vi "live open.vi"(8 "error in (no error)":errorcluster, 11 "DAQCascade512II":refnum<class "DAQCascade512II.lvclass">) -> (0 "error out":errorcluster, 3 "DAQCascade512II out":refnum<class "DAQCascade512II.lvclass">)   [LabVIEW 2012, in "DAQCascade512II.lvclass"]
uses:
  DAQCascade512II.lvclass
  DAQCascade512II.lvclass/DAQCascade512II.ctl
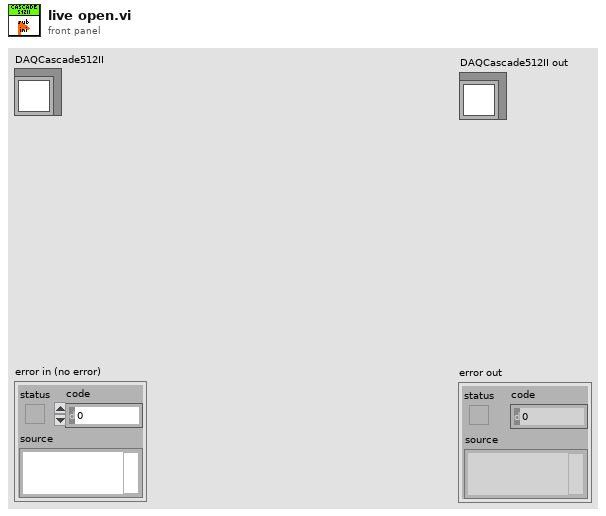
[diagram p1: front panel]
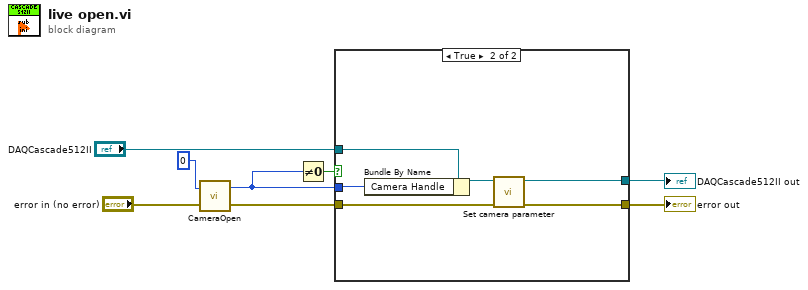
[diagram p0: block diagram]
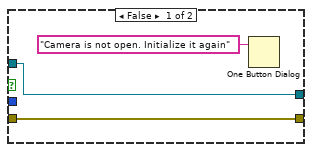
[diagram p2: hidden frame]
diagram:
  n1 = call <userlib>:"CameraOpen.vi"("error in"="error in (no error)", "Camera Device ID"=u32 0) -> ("error out"=w3:errorcluster, "Camera Handle"=w1:u32)
  n2 = Not Equal To 0?(x=w1) -> (x != 0?=w2:bool)
  n3 = case shown="True" w2 {
    tunnel: [w9 w13] -> w7
    tunnel: [w11 w12] -> w8
    tunnel: w1 -> [_ w17]
    tunnel: "DAQCascade512II" -> [w11 w16]
    tunnel: w3 -> [w9 w14]
    frame False {
      n4 = One Button Dialog(message="Camera is not open. Initialize it again") -> ()  [unwired: 1 in, 1 out]
    }
    frame True {
      n5 = Bundle By Name(cluster=w16, "Camera Handle"=w17) -> (w15:refnum<class "DAQCascade512II.lvclass">)
      n6 = call-dynamic "Set camera parameter.vi"("error in (no error)"=w14, "DAQCascade512II in"=w15) -> ("error out"=w13:errorcluster, "DAQCascade512II out"=w12:refnum<class "DAQCascade512II.lvclass">)  [unwired: 8 in]
    }
  }
  "error out" <- w7
  "DAQCascade512II out" <- w8
